vi "Subvi gating out.vi"(10 "Memory label":refnum<k21>="Pixel sync buffer") -> ()   [LabVIEW 2017]
uses:
  <vilib>/rvi/DataTransferAndStorage/Container/Common/niFpgaContainerExecOnDevCompGetState.vi
  <vilib>/rvi/Emulation/niFpgaEmulationIsFPGAContextNoSignature.vi
  <vilib>/rvi/DataTransferAndStorage/Container/Common/niFpgaContainerGetUniqueNameForEmu.vi
  <vilib>/rvi/Emulation/niFpgaProcessEmulError.vi
  <vilib>/rvi/Emulation/niFpgaSctlEmulationGetInTimedLoop.vi
  <vilib>/rvi/errors/nirviReportUnexpectedCaseInternalError (U32).vi
  <vilib>/rvi/Memory/Memory_Emulation/niFpgaMemoryEmulationCacheClearOnFirstRun.vi
  <vilib>/rvi/Memory/Memory_Emulation/nirvimemoryEmulationManagerCache_MakeExclusive.vi
  <vilib>/rvi/Memory/Memory_Emulation/niFpgaMemoryEmulationValidateCache.vi
  <vilib>/rvi/Memory/Memory_Emulation/nirvimemoryEmulationManagerCache_InsertValue.vi
  <vilib>/Utility/error.llb/Clear Errors.vi
  <vilib>/rvi/Memory/Memory_Emulation/nirvimemoryEmulationManagerCache_ReleaseExclusive.vi
  <vilib>/rvi/Memory/Memory_Emulation/nirvimemoryEmulationManagerCache_GetValue.vi
  <vilib>/rvi/Memory/Memory_Emulation/nirvimemoryEmulationManagerCache_SetValue.vi
  <vilib>/rvi/Emulation/niFpgaSctlEmulationResourceMgr.vi
  GV pixel sync.vi
  <vilib>/rvi/DataTransferAndStorage/Container/XNode/niFpgaContainer.xnode
  <vilib>/rvi/Memory/Memory_Emulation/niFpgaMemoryEmulationRefIn.vi
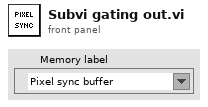
[diagram p1: front panel]
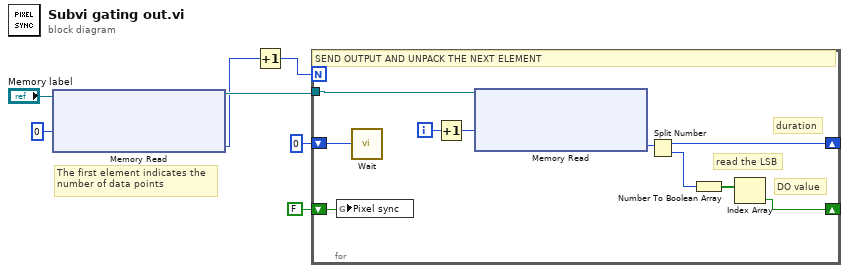
[diagram p0: block diagram]
diagram:
  # "The first element indicates the\nnumber of data points"
  n1 = xnode ("Memory Read")("Address"=u32 0, "Memory In"="Memory label") -> ("Data"=w5:u32, "Memory Out"=w7:refnum<k21>)
  n2 = Increment(x=w5) -> (x+1=w6:u32)
  n3 = for {
    N: w6 -> [_]
    shift-right: [w12] -> _
    shift-left: FALSE -> [w8]
    shift-right: [w14] -> _
    shift-left: u16 0 -> [w13]
    tunnel: w7 -> [w9]
    i -> [w11]
    # "read the LSB"
    # "DO value"
    # "duration"
    # "SEND OUTPUT AND UNPACK THE NEXT ELEMENT"
    n4 = global write "GV pixel sync.vi" "Pixel sync"(w8) -> ()
    n5 = call "Wait"("Count(Ticks)"=w13) -> ()  [unwired: 1 out]
    n6 = Increment(x=w11) -> (x+1=w10:i32)
    n7 = xnode ("Memory Read")("Address"=w10, "Memory In"=w9) -> ("Data"=w16:u32)  [unwired: 1 out]
    n8 = Split Number(x=w16) -> (hi(x)=w14:u16, lo(x)=w15:u16)
    n9 = Number To Boolean Array(number=w15) -> (Boolean array=w17:bool[])
    n10 = Index Array(array=w17) -> (element=w12:bool)  [unwired: 1 in]
  }
